vi "setup.vi"(8 "error in":errorcluster) -> (0 "error out":errorcluster, 2 "detector-lines":T1, 3 "Source Out":dbl[][](array[numeric]))   [LabVIEW 2023]
panel:
  out "Detector Out":dbl[][](array[numeric])
  out "led detector":bool
  out "led source":bool
  in  "source":bool
  in  "det":bool
  in  "Stop":bool
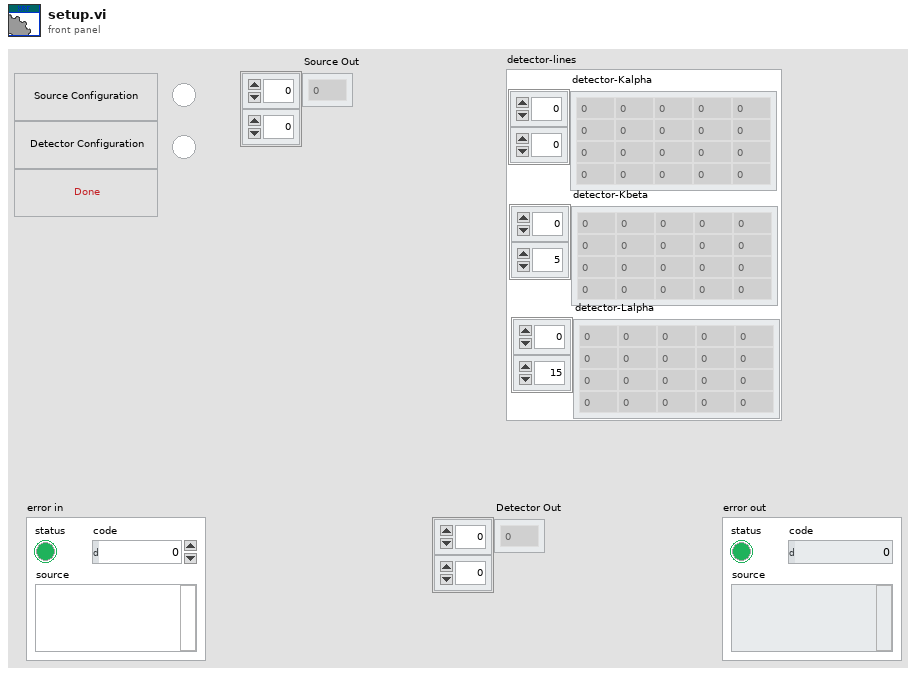
[diagram p1: front panel]
types:
  T1 = cluster{"detector-Kalpha":dbl[][], "detector-Kbeta":dbl[][], "detector-Lalpha":dbl[][]}
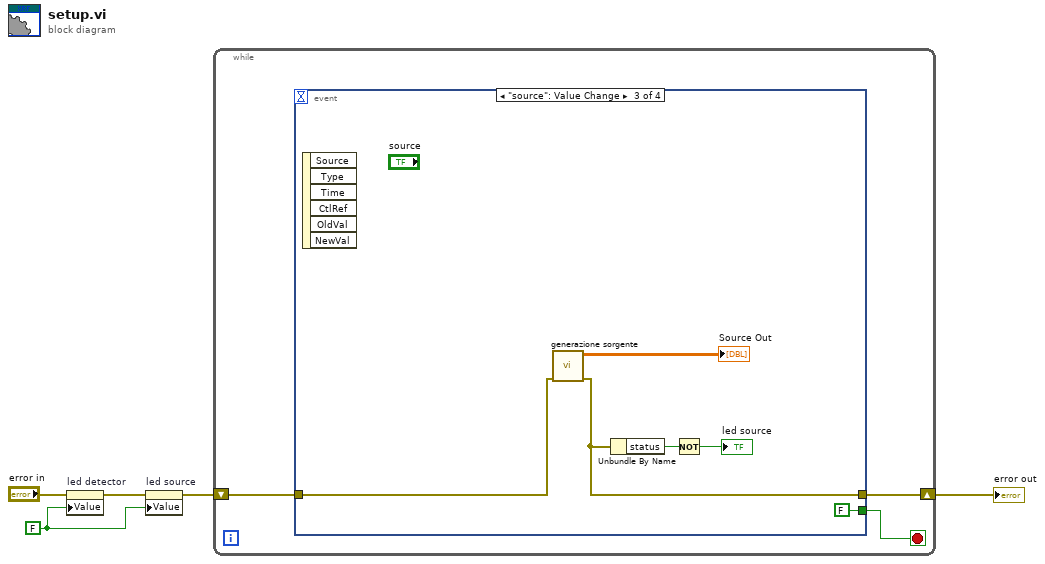
[diagram p0: block diagram]
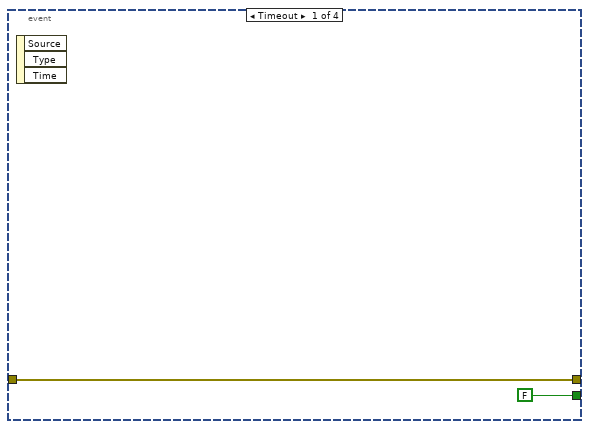
[diagram p2: hidden frame]
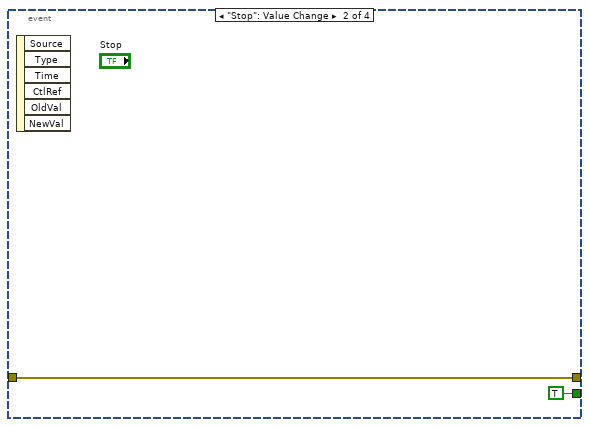
[diagram p3: hidden frame]
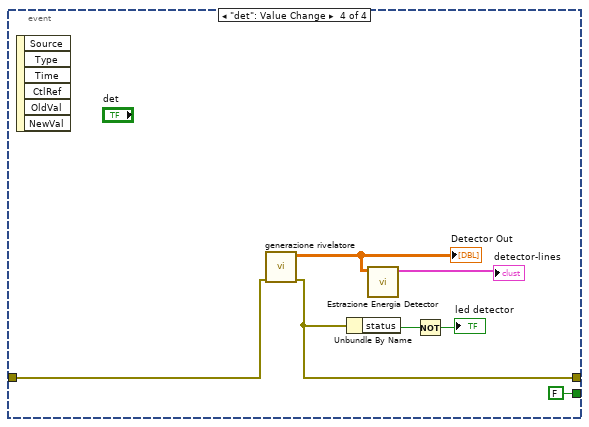
[diagram p4: hidden frame]
diagram:
  w1 = FALSE
  n1 = property on="led detector" class="Bool (strict)"(error in="error in", "Value"=w1) -> (error out=w3:errorcluster)  [unwired: 1 in, 1 out]
  n2 = property on="led source" class="Bool (strict)"(error in=w3, "Value"=w1) -> (error out=w2:errorcluster)  [unwired: 1 in, 1 out]
  n3 = while {
    shift-right: [w7] -> w5
    shift-left: w2 -> [w8]
    stop <- w6 stop-if-true
    n4 = event shown="[2] \"source\": Value Change" {
      selector: _ -> [_ _ _ _]
      dyn-events: _ -> [_ _ _ _]
      timeout: _ -> [_ _ _ _]
      tunnel: w8 -> [w10 w12 w17 w24]
      tunnel: [w10 w12 w16 w23] -> w7
      tunnel: [FALSE TRUE FALSE FALSE] -> w6
      event Timeout {
        n5 = event-data() -> ()  [unwired: 1 in, 3 out]
      }
      event "Stop": Value Change {
        n6 = event-data() -> ()  [unwired: 1 in, 6 out]
      }
      event "source": Value Change {
        n7 = event-data() -> ()  [unwired: 1 in, 6 out]
        n8 = call "generazione sorgente.vi"("error in"=w17) -> ("error out"=w16:errorcluster, "Source Out"=→"Source Out":dbl[][])  [unwired: 9 in]
        n9 = Unbundle By Name(w16) -> ("status"=w15:bool)
        n10 = Not(x=w15) -> (.not. x?=→"led source":bool)
      }
      event "det": Value Change {
        n11 = event-data() -> ()  [unwired: 1 in, 6 out]
        n12 = call "generazione rivelatore.vi"("error in"=w24) -> ("error out"=w23:errorcluster, "Detector Out"=w20:dbl[][])  [unwired: 9 in]
        "Detector Out" <- w20
        n13 = Unbundle By Name(w23) -> ("status"=w21:bool)
        n14 = call "Estrazione Energia Detector.vi"("Detector In"=w20) -> ("detector-lines"=→"detector-lines":T1)  [unwired: 10 in]
        n15 = Not(x=w21) -> (.not. x?=→"led detector":bool)
      }
    }
  }
  "error out" <- w5
